vi "PUSH (SubVI).vi"(6 "Push Time":dbl=5.0 caption="Delay Time (s)", 11 "Digital I/O Pin":u8=7) -> (7 "Arduino Resource":T1={"VISA resource"="COM3", "Board Type"=enum."Uno", "Connection Type"=enum."USB / Serial", "Bytes Per Packet (15)"=15})   [LabVIEW 2016]
uses:
  <vilib>/LabVIEW Interface for Arduino/Type Defs/Arduino Resource.ctl
  <vilib>/LabVIEW Interface for Arduino/Type Defs/Board Type.ctl
  <vilib>/LabVIEW Interface for Arduino/Type Defs/Pin Mode.ctl
  <vilib>/LabVIEW Interface for Arduino/LabVIEW Interface for Arduino.lvlib
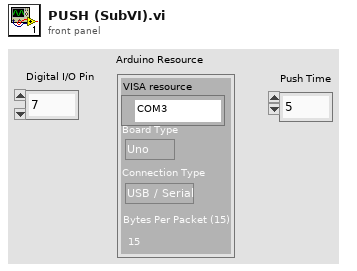
[diagram p1: front panel]
types:
  T1 = typedef "LabVIEW Interface for Arduino.lvlib/Arduino Resource.ctl" = cluster{"VISA resource":refnum<visa-resource-name>, "Board Type":T2, "Connection Type":enum8{"USB / Serial"}, "Bytes Per Packet (15)":u8}
  T2 = typedef "LabVIEW Interface for Arduino.lvlib/Board Type.ctl" = enum16{"Uno", "Dimuelanove w/Atmega 328", "Mega 2560"}
  T3 = typedef "LabVIEW Interface for Arduino.lvlib/Pin Mode.ctl" = enum8{"Input", "Output"}
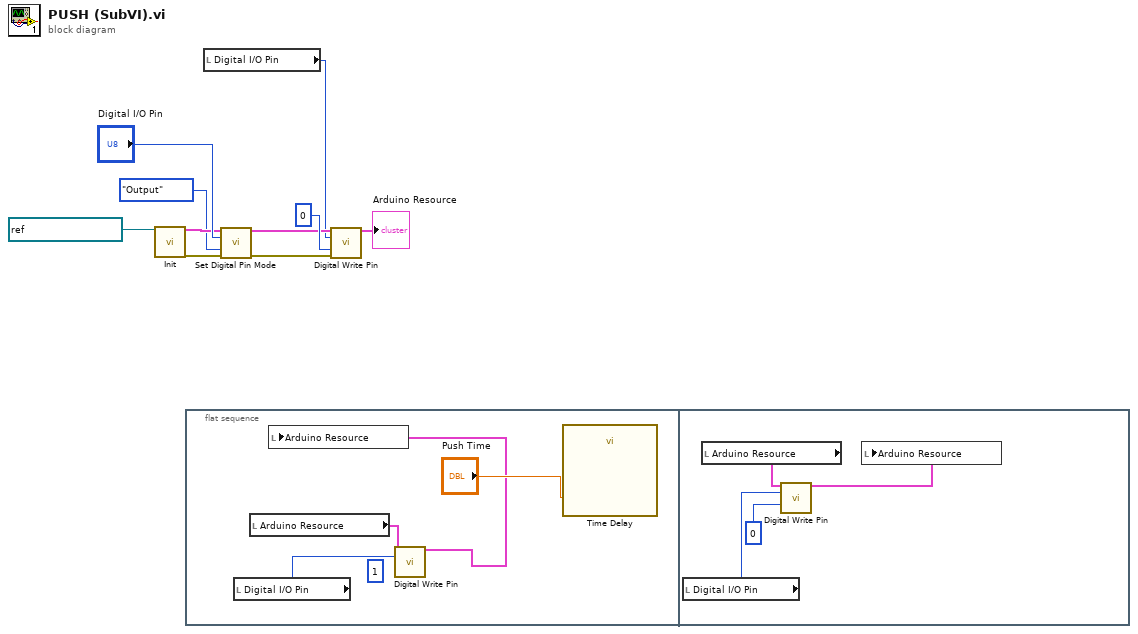
[diagram p0: block diagram]
diagram:
  n1 = call <vilib>:"Init.vi"("VISA resource"=refnum<visa-resource-name> "COM3") -> ("Arduino Resource"=w5:T1, "error out"=w3:errorcluster)  [unwired: 17 in]
  n2 = flat-sequence {
    frame #0 {
      (unwired) u8 1 ("Value (0)")
      n3 = local read "Digital I/O Pin"() -> (w11:u8)
      n4 = local read "Arduino Resource"() -> (w12:T1)
      n5 = call <vilib>:"Digital Write Pin.vi"("Arduino Resource"=w12, "Digital I/O Pin (0)"=w11) -> ("Arduino Resource"=w13:T1)  [unwired: 12 in, 1 out]
      n6 = local write "Arduino Resource"(w13) -> ()
      n7 = call "Time Delay"("Delay Time (s)"="Push Time") -> ()  [unwired: 10 in, 1 out]
    }
    frame #1 {
      n8 = local read "Digital I/O Pin"() -> (w17:u8)
      n9 = local read "Arduino Resource"() -> (w16:T1)
      n10 = call <vilib>:"Digital Write Pin.vi"("Arduino Resource"=w16, "Digital I/O Pin (0)"=w17, "Value (0)"=u8 0) -> ("Arduino Resource"=w15:T1)  [unwired: 11 in, 1 out]
      n11 = local write "Arduino Resource"(w15) -> ()
    }
  }
  n12 = local read "Digital I/O Pin"() -> (w1:u8)
  n13 = call <vilib>:"Set Digital Pin Mode.vi"("Arduino Resource"=w5, "Digital I/O Pin"="Digital I/O Pin", "Pin Mode (Input)"=Pin_Mode."Output", "error in"=w3) -> ("Arduino Resource"=w7:T1, "error out"=w8:errorcluster)  [unwired: 10 in]
  n14 = call <vilib>:"Digital Write Pin.vi"("Arduino Resource"=w7, "Digital I/O Pin (0)"=w1, "Value (0)"=u8 0, "error in"=w8) -> ("Arduino Resource"=→"Arduino Resource":T1)  [unwired: 10 in, 1 out]
